vi "Generate Name Prefixes.vi"(8 "error in":errorcluster, 9 "Add Prefix?":bool=TRUE, 10 "Container - Regex pairs":T1=[{"Container to create"="TEST", "Regex"="^test_.*\\.vi"}, {"Container to create"="TEST", "Regex"="_test.vi$"}, {"Container to create"="DRV", "Regex"="^DRV_.*\\.lv.*$"}, {"Container to create"="HWT", "Regex"="^HWT_.*\\.lv.*$"}, {"Container to create"="FCN", "Regex"="^FCN_.*\\.lv.*$"}, {"Container to create"="INS", "Regex"="^INS_.*\\.lv.*$"}], 11 "Dep Names and Paths":T2) -> (0 "error out":errorcluster, 3 "Prefixed Dep Names and Paths":T2)   [LabVIEW 2018, in "Shared Dependencies.lvlib"]
uses:
  Shared Dependencies/Shared Dependencies.lvlib
  Dep Names and Paths.ctl
  Shared Dependencies/Container - Regex array.ctl
  Name and Dependency Processing.lvlib
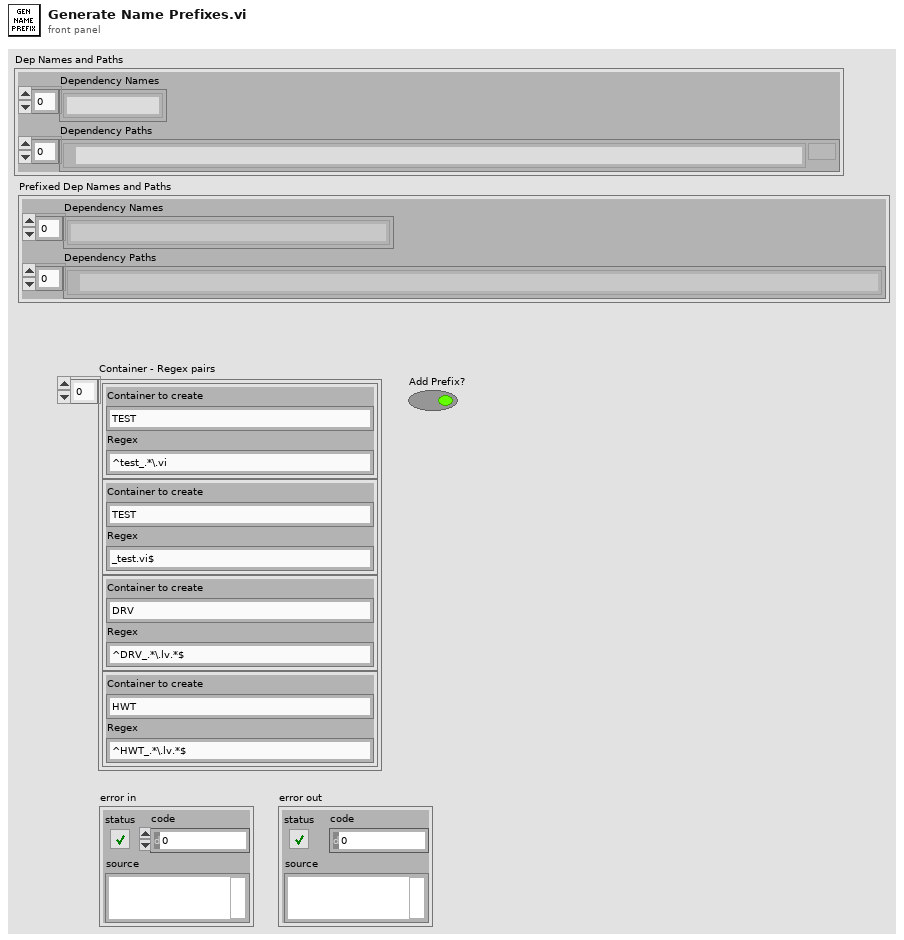
[diagram p1: front panel]
types:
  T1 = typedef "Shared Dependencies.lvlib/Container - Regex array.ctl" = cluster{"Container to create":string, "Regex":string}[]
  T2 = typedef "Name and Dependency Processing.lvlib/Dep Names and Paths.ctl" = cluster{"Dependency Names":string[], "Dependency Paths":path[]}
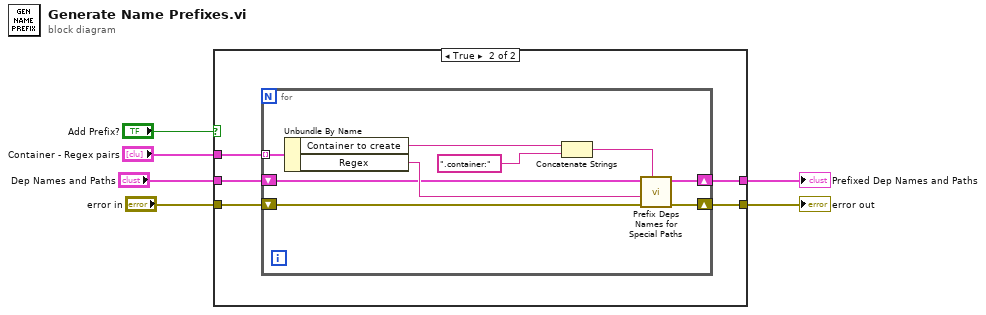
[diagram p0: block diagram]
diagram:
  n1 = case shown="True" "Add Prefix?" {
    tunnel: [w8 w13] -> w6
    tunnel: [w7 w12] -> w5
    tunnel: "Container - Regex pairs" -> [_ w11]
    tunnel: "Dep Names and Paths" -> [w8 w10]
    tunnel: "error in" -> [w7 w9]
    frame False {
    }
    frame True {
      n2 = for {
        tunnel: w11 -> [w20] mode=indexing
        shift-right: [w22] -> w13
        shift-left: w10 -> [w18]
        shift-right: [w21] -> w12
        shift-left: w9 -> [w17]
        n3 = Unbundle By Name(w20) -> ("Container to create"=w16:string, "Regex"=w19:string)
        n4 = Concatenate Strings(w16, ".container:" ("string")) -> (w14:string)
        n5 = call "Prefix Deps Names for Special Paths.vi"("Prefix to add"=w14, "error in"=w17, "Regex to identify need for prefix"=w19, "Dep Names and Paths"=w18) -> ("error out"=w21:errorcluster, "Prefixed Dep Names and Paths"=w22:T2)  [unwired: 6 in]
      }
    }
  }
  "Prefixed Dep Names and Paths" <- w6
  "error out" <- w5
